vi "Process.vi"(8 "error in (no error)":errorcluster, 10 "Results Notifier":refnum<notifier>, 11 "ReadCommand in":refnum<class "ReadCommand.lvclass">) -> (0 "error out":errorcluster, 3 "ReadCommand out":refnum<class "ReadCommand.lvclass">)   [LabVIEW 2023, in "HAF.lvlib" / "ReadCommand.lvclass"]
doc: "Processes the Write Command against the specified Driver for the Command.\n\nThe Driver will ensure it is initialised and process the Command Settings; it is responsible for interacting with the Instrument.\n\nAny Results Notifier passed is ignored by a Write Command, because no result is processed. It may be used by a Read Command."
uses:
  ReadCommand.lvclass
  ReadCommand.lvclass/ReadCommand.ctl
  WriteCommand/WriteCommand.lvclass
  Driver/Driver.lvclass
  \\Mac\Home/Documents/LabVIEW Data/ProjectTemplates/Source/HAF/WriteCommand/WriteCommand.lvclass
  \\Mac\Home/Documents/LabVIEW Data/ProjectTemplates/Source/HAF/Executable/Executable.lvclass
  \\Mac\Home/Documents/LabVIEW Data/ProjectTemplates/Source/HAF/ReadCommand/ReadCommand.lvclass
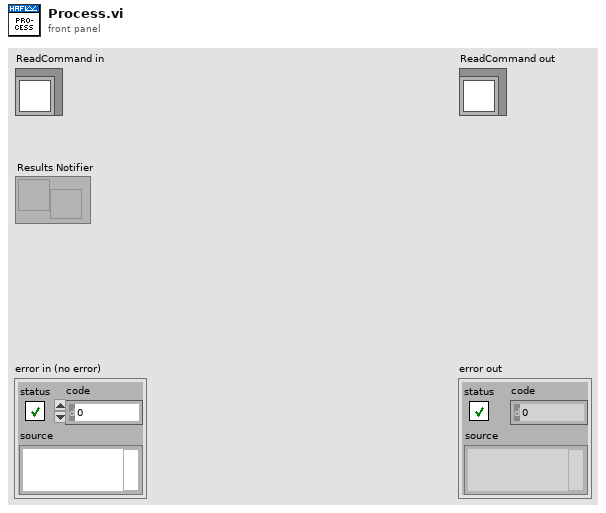
[diagram p1: front panel]
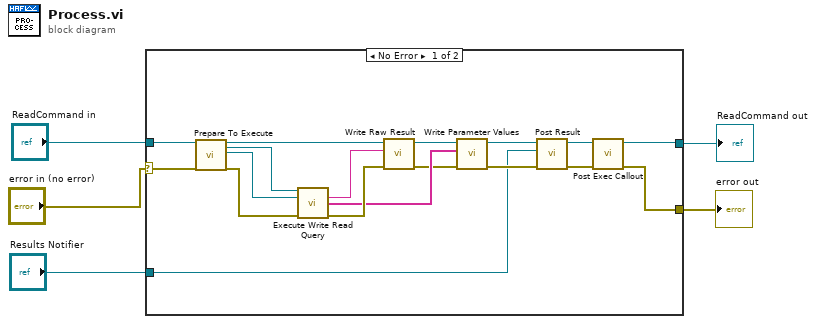
[diagram p0: block diagram]
diagram:
  n1 = case shown="No Error" "error in (no error)" {
    selector: "error in (no error)" -> [w10 w24]
    tunnel: "ReadCommand in" -> [w11 w25]
    tunnel: "Results Notifier" -> [w16 _]
    tunnel: [w13 w25] -> w2
    tunnel: [w12 w24] -> w1
    frame No Error {
      n2 = call "Prepare To Execute.vi"("WriteCommand in"=w11, "error in (no error)"=w10) -> ("WriteCommand out"=w9:refnum<class "ReadCommand.lvclass">, "Driver out"=w8:refnum<class "Driver.lvclass">, "Executable"=w7:refnum<class "Executable.lvclass">, "error out"=w6:errorcluster)  [unwired: 14 in]
      n3 = call-dynamic "Execute Write Read Query.vi"("Driver in"=w8, "Executable In"=w7, "error in (no error)"=w6) -> ("Raw Result"=w23:string, "Raw Parameter Results"=w20:string[], "error out"=w22:errorcluster)  [unwired: 8 in, 2 out]
      n4 = call-dynamic "Write Raw Result.vi"("error in (no error)"=w22, "Raw Result"=w23, "ReadCommand in"=w9) -> ("error out"=w19:errorcluster, "ReadCommand out"=w21:refnum<class "ReadCommand.lvclass">)  [unwired: 7 in]
      n5 = call-dynamic "Write Parameter Values.vi"("error in (no error)"=w19, "Parameter Values"=w20, "WriteCommand in"=w21) -> ("error out"=w17:errorcluster, "WriteCommand out"=w18:refnum<class "ReadCommand.lvclass">)  [unwired: 7 in]
      n6 = call-dynamic "Post Result.vi"("error in (no error)"=w17, "Results Notifier"=w16, "ReadCommand in"=w18) -> ("error out"=w14:errorcluster, "ReadCommand out"=w15:refnum<class "ReadCommand.lvclass">)  [unwired: 7 in]
      n7 = call-dynamic "Post Exec Callout.vi"("error in (no error)"=w14, "WriteCommand in"=w15) -> ("error out"=w12:errorcluster, "WriteCommand out"=w13:refnum<class "ReadCommand.lvclass">)  [unwired: 8 in]
    }
    frame Error {
    }
  }
  "error out" <- w1
  "ReadCommand out" <- w2
